vi "final shn 2 .vi"() -> ()   [LabVIEW 2018]
doc: "The myRIO Project template acquires acceleration data from the onboard accelerometer and displays the changes of acceleration values in a waveform chart."
uses:
  <vilib>/myRIO/Instrument Drivers/Onboard IO/DIO/typedefs/DIO Reference.ctl
  <vilib>/myRIO/Common/Instrument Driver Framework/Utilities/typedefs/myRIO Generic Hardware Reference.ctl
  <vilib>/myRIO/Common/Instrument Driver Framework/Utilities/typedefs/Hardware Version Enum.ctl
  <vilib>/myRIO/Common/Instrument Driver Framework/Utilities/typedefs/myRIO v1.0 Reference.ctl
  <vilib>/myRIO/Common/Instrument Driver Framework/Utilities/typedefs/Generic FPGA Reference.ctl
  <vilib>/myRIO/Common/Instrument Driver Framework/myRIO v1.0/DIO/typedefs/DIO Channels List.ctl
  <vilib>/myRIO/Common/Instrument Driver Framework/myRIO v1.0/DIO/typedefs/DIO Channels Enum.ctl
  <vilib>/userdefined/High Color/nirio_resource_hc.ctl
  <vilib>/myRIO/Instrument Drivers/Onboard IO/PWM/typedefs/PWM Reference.ctl
  <vilib>/myRIO/Common/Instrument Driver Framework/myRIO v1.0/PWM/typedefs/PWM Channels Enum.ctl
  <vilib>/myRIO/Instrument Drivers/Onboard IO/PWM/typedefs/PWM Configuration.ctl
  <vilib>/myRIO/Common/Instrument Driver Framework/Utilities/vis/Is FPGA Ref Available.vi
  <vilib>/myRIO/Common/Instrument Driver Framework/myRIO v1.0/DIO/vis/myRIO v1.1 Open DIO.vi
  <vilib>/myRIO/Instrument Drivers/Onboard IO/DIO/vis/Write.vi
  <vilib>/myRIO/Common/Instrument Driver Framework/myRIO v1.0/PWM/vis/myRIO v1.1 Open PWM.vi
  <vilib>/myRIO/Instrument Drivers/Onboard IO/PWM/vis/Set Duty Cycle and Frequency.vi
  <vilib>/myRIO/Common/Instrument Driver Framework/Utilities/vis/Validate Channels.vi
  <vilib>/myRIO/Common/Instrument Driver Framework/myRIO v1.0/DIO/vis/myRIO v1.0 Reserve DIO.vi
  <vilib>/myRIO/Common/Instrument Driver Framework/myRIO v1.0/PWM/vis/myRIO v1.0 Reserve PWM.vi
  <vilib>/myRIO/Common/Instrument Driver Framework/myRIO v1.0/Resource Manager/vis/myRIO v1.0 Reserve Channel List.vi
  <vilib>/myRIO/Common/Instrument Driver Framework/myRIO v1.0/DIO/vis/myRIO v1.0 Build MUX Configuration DIO.vi
  <vilib>/myRIO/Common/Instrument Driver Framework/myRIO v1.0/PWM/vis/myRIO v1.0 Build MUX Configuration PWM.vi
  <vilib>/myRIO/Common/Instrument Driver Framework/myRIO v1.0/Resource Manager/vis/myRIO v1.0 Reserve Channel.vi
  <vilib>/myRIO/Common/Instrument Driver Framework/myRIO v1.0/Resource Manager/vis/myRIO v1.0 Unreserve Channel.vi
  <vilib>/myRIO/Common/Instrument Driver Framework/myRIO v1.0/Resource Manager/vis/myRIO v1.0 Create Configuration List.vi
  <vilib>/myRIO/Common/Instrument Driver Framework/myRIO v1.0/Resource Manager/vis/myRIO v1.0 Build Mutex Name.vi
  <vilib>/Utility/VariantDataType/GetNumericInfo.vi
  <vilib>/Utility/error.llb/Error Cluster From Error Code.vi
  <vilib>/myRIO/Common/Instrument Driver Framework/myRIO v1.0/myRIO v1.1 Open.vi
  <vilib>/myRIO/Common/Instrument Driver Framework/Utilities/vis/IO Manager.vi
  <vilib>/myRIO/Common/Instrument Driver Framework/Utilities/vis/Configuration Manager.vi
  <vilib>/myRIO/Common/Instrument Driver Framework/myRIO v1.0/Resource Manager/vis/myRIO v1.0 Configure IO.vi
  <vilib>/myRIO/Common/Instrument Driver Framework/myRIO v1.0/myRIO v1.0 Close.vi
  <vilib>/myRIO/Common/Instrument Driver Framework/myRIO v1.0/DIO/vis/myRIO v1.0 Write DIO.vi
  <vilib>/myRIO/Common/Instrument Driver Framework/myRIO v1.0/PWM/vis/myRIO v1.0 Write PWM.vi
  <vilib>/myRIO/Express VI/Onboard Devices/LED/LED Express VI.xnode
  <vilib>/myRIO/Instrument Drivers/Onboard IO/DIO/vis/myRIO DIO Open.xnode
  <vilib>/myRIO/Express VI/Onboard IO/PWM/PWM Express VI.xnode
  <vilib>/myRIO/Instrument Drivers/Onboard IO/PWM/vis/myRIO PWM Open.xnode
  <vilib>/myRIO/Express VI/Onboard IO/DO/DO Express VI.xnode
  <vilib>/myRIO/Instrument Drivers/Onboard IO/PWM/PWM.lvlib
  <vilib>/myRIO/Instrument Drivers/Onboard IO/DIO/DIO.lvlib
panel:
  in  "left":bool
  in  "Right":bool
  out "jot connection":bool
  in  "Stop Button 2":bool
  out "message from rio 2":string[](array[string])
  out "Boolean 4":bool=TRUE
  out "Boolean 3":bool=TRUE
  out "Boolean 2":bool
  in  "Stop":bool
  out "Message from Ground Station":string[](array[string])
  in  "horn":bool
  in  "CUTOUT":bool
  in  "Red":bool
  in  "Green":bool
  in  "Yellow":bool
  out "yaw left":bool
  out "yaw right":bool
  out "Duty Cycle 2":dbl=0.5
  out "Duty Cycle":dbl=0.5
  out "thruster 22":dbl
  out "thruster 11":dbl
  out "thruster 2":dbl(slide) scale=0.44..0.76
  out "thruster 1":dbl(slide) scale=0.44..0.76
  out "message from rio":string[](array[string])
  out "surv":dbl
  out "yav":dbl
  out "yad":dbl
  out "surd":dbl
  in  "Stop Button":bool
  out "speed":dbl(slide) scale=0.5..1.0
  out "yaw":dbl(slide) scale=0.0..10000.0
  out "surge":dbl(slide) scale=0.0..10000.0
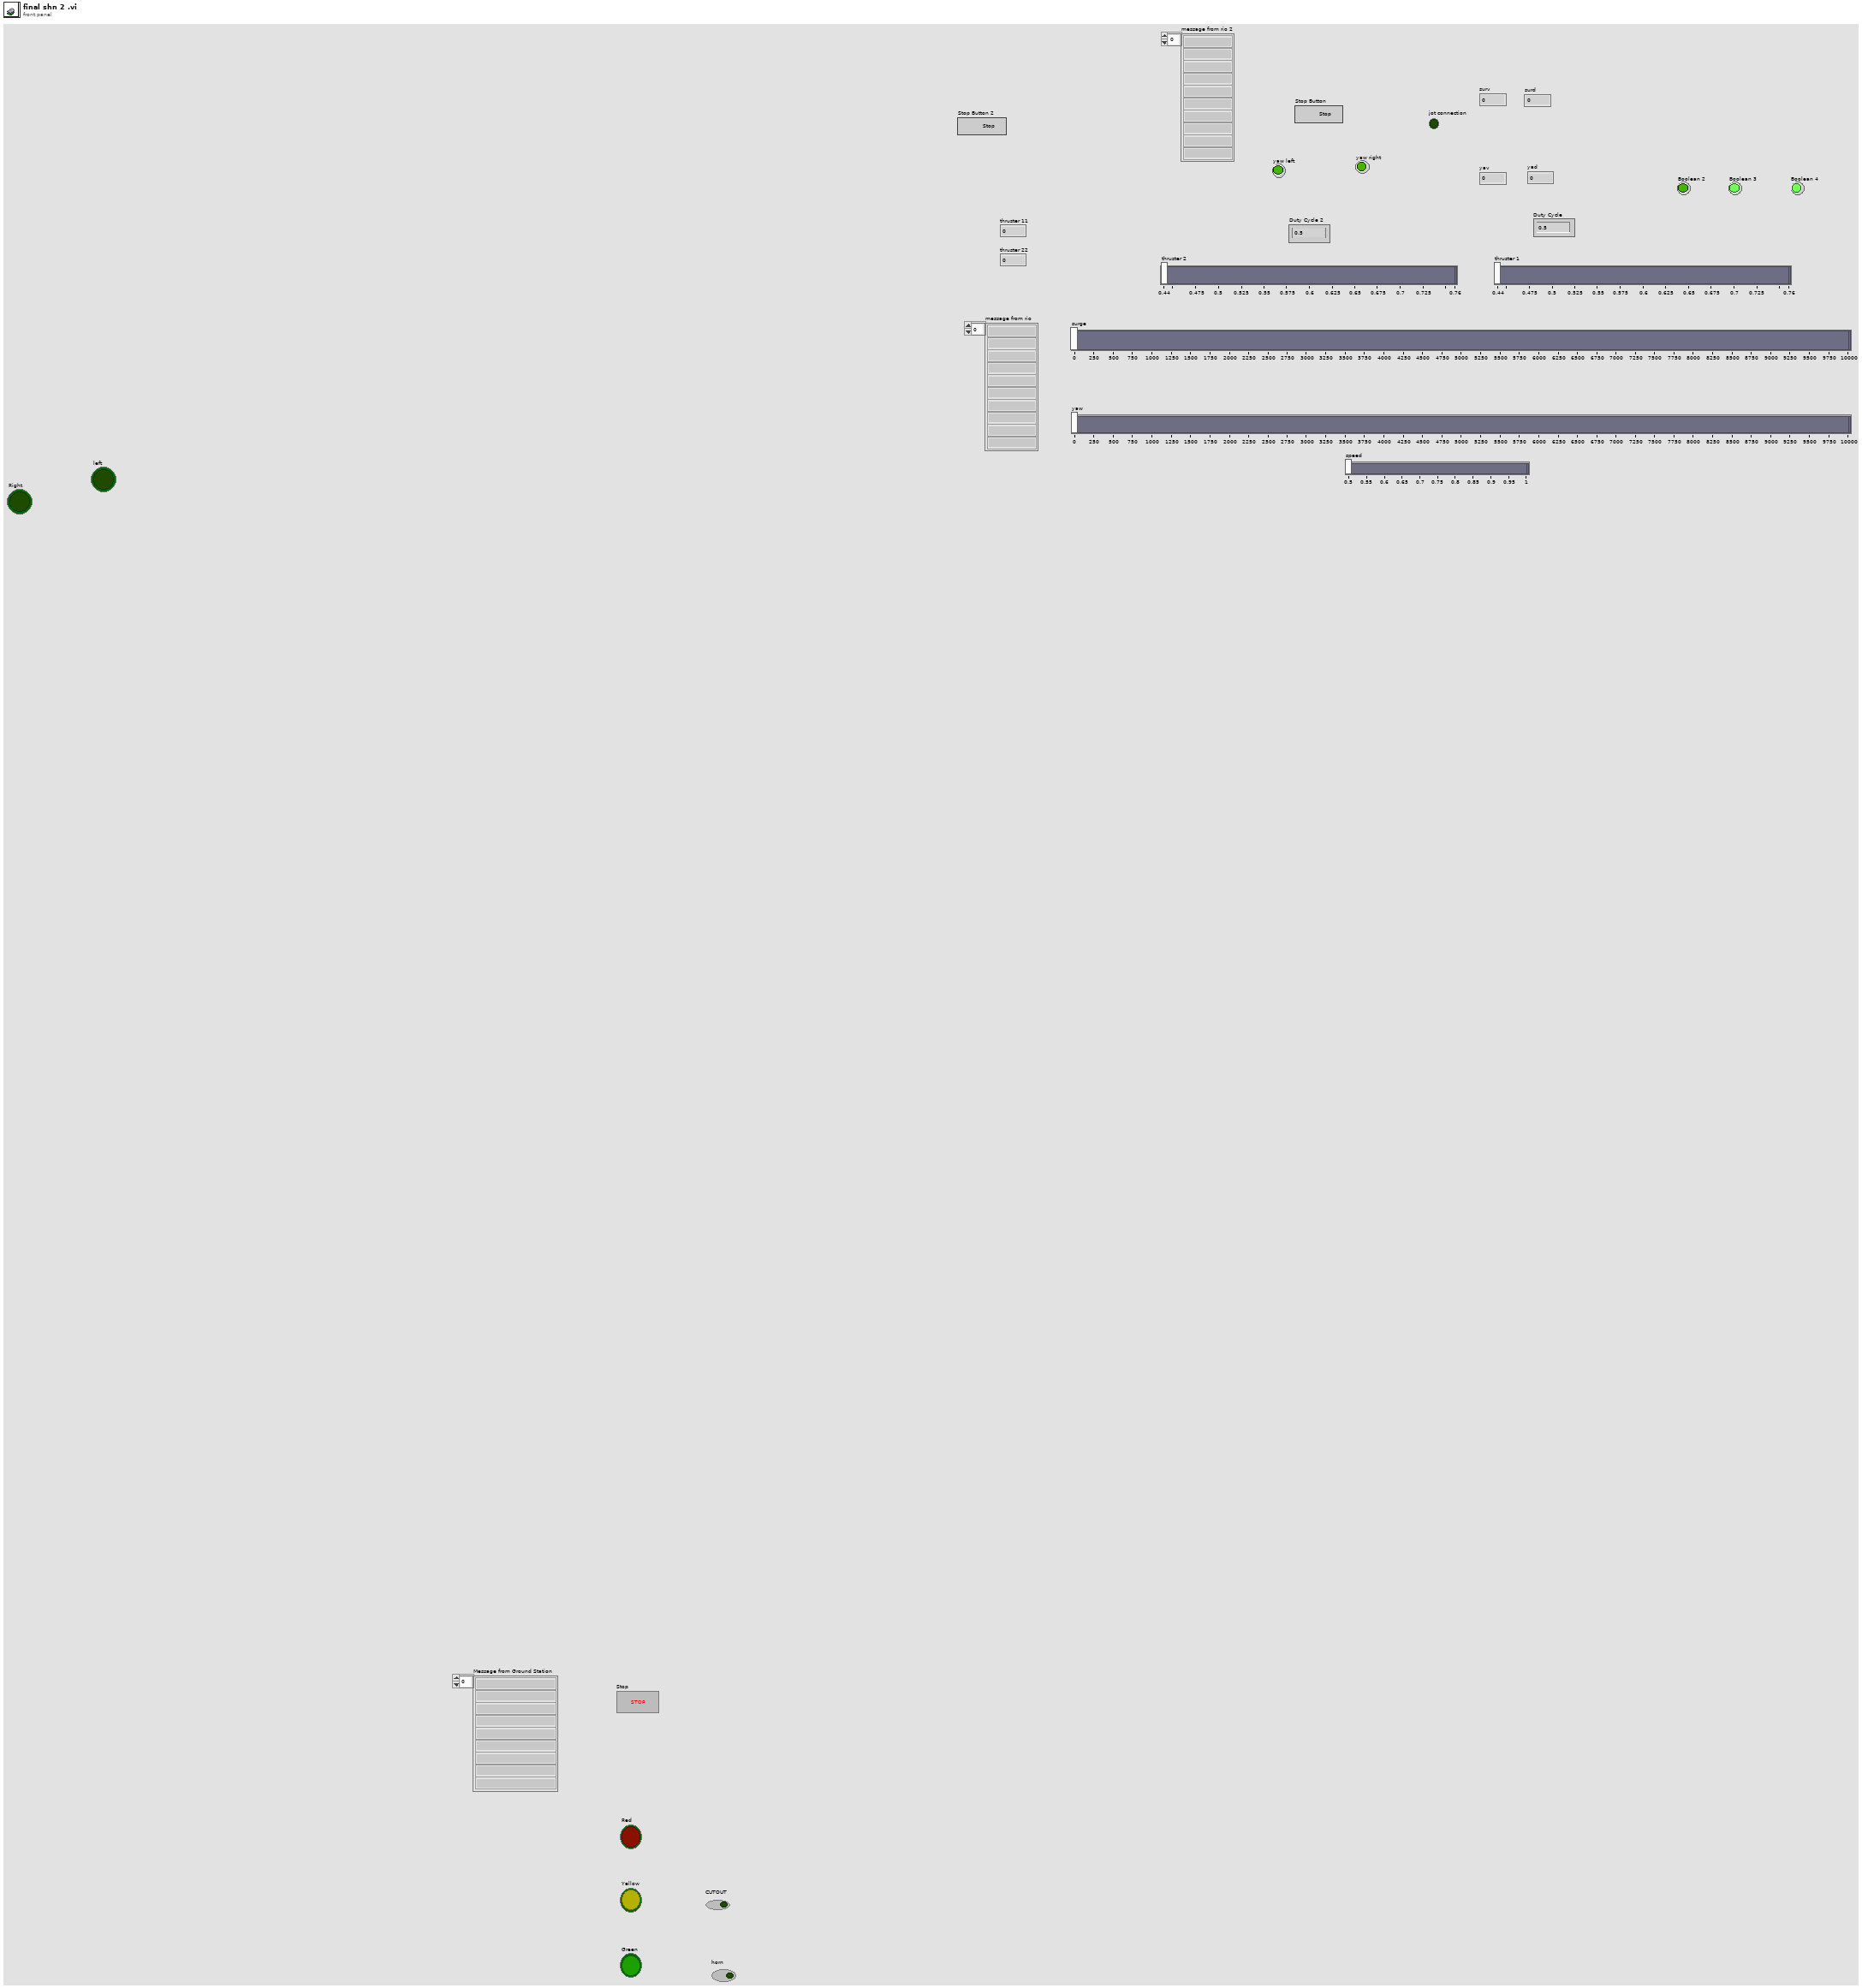
[diagram p1: front panel]
types:
  T1 = typedef "DIO.lvlib/DIO Reference.ctl" = cluster{"myRIO Reference":T2, "DIO Channels List":T6}
  T2 = typedef "myRIO Generic Hardware Reference.ctl" = cluster{"myRIO Model":T3, "myRIO Hardware Reference":T4}
  T3 = typedef "Hardware Version Enum.ctl" = enum16{"Unknown", "myRIO-1900", "myRIO-1950", "roboRIO", "NI ELVIS RIO CM", "ELVIS III"}
  T4 = typedef "myRIO v1.0 Reference.ctl" = cluster{"Generic FPGA Reference":T5, "Allow multiple opens":bool}
  T5 = typedef "Generic FPGA Reference.ctl" = refnum<k20>
  T6 = typedef "DIO Channels List.ctl" = T7[]
  T7 = typedef "DIO Channels Enum.ctl" = enum16{"Not Connected", "C/DIO0", "C/DIO1", "C/DIO2", "C/DIO3", "C/DIO4", "C/DIO5", "C/DIO6", "C/DIO7", "A/DIO0", "A/DIO1", "A/DIO2", "A/DIO3", "A/DIO4", "A/DIO5", "A/DIO6", "A/DIO7", "A/DIO8", "A/DIO9", "A/DIO10", "A/DIO11", "A/DIO12", "A/DIO13", "A/DIO14", "A/DIO15", "A/DIO16", "A/DIO17", "A/DIO18", "A/DIO19", "B/DIO0", "B/DIO1", "B/DIO2", "B/DIO3", "B/DIO4", "B/DIO5", "B/DIO6", "B/DIO7", "B/DIO8", "B/DIO9", "B/DIO10", "B/DIO11", "B/DIO12", "B/DIO13", "B/DIO14", "B/DIO15", "B/DIO16", "B/DIO17", "B/DIO18", "B/DIO19", "LED0", "LED1", "LED2", "LED3", "Button0", "DIO/DIO0", "DIO/DIO1", "DIO/DIO2", "DIO/DIO3", "DIO/DIO4", "DIO/DIO5", "DIO/DIO6", "DIO/DIO7", "DIO/DIO8", "DIO/DIO9", "SPI/CS0", "SPI/CS1", "SPI/CS2", "SPI/CS3", "LED RADIO (Green)", "LED RADIO (Red)", "LED COMM (Green)", "LED COMM (Red)", "LED MODE (Green)", "LED MODE (Red)"}
  T8 = typedef "nirio_resource_hc.ctl" = tag
  T9 = cluster{"[0]":string, "[1]":string, "[2]":string, "[3]":string, "[4]":string, "[5]":string, "[6]":string, "[7]":string, "[8]":string}
  T10 = typedef "PWM.lvlib/PWM Reference.ctl" = cluster{"myRIO Reference":T2, "PWM Channels Enum":T11, "PWM Configuration":T12}
  T11 = typedef "PWM Channels Enum.ctl" = enum16{"Not Connected", "C/PWM0", "C/PWM1", "A/PWM0", "A/PWM1", "A/PWM2", "A/PWM3", "A/PWM4", "A/PWM5", "A/PWM6", "A/PWM7", "A/PWM8", "A/PWM9", "A/PWM10", "A/PWM11", "A/PWM12", "A/PWM13", "A/PWM14", "A/PWM15", "A/PWM16", "A/PWM17", "A/PWM18", "A/PWM19", "B/PWM0", "B/PWM1", "B/PWM2", "B/PWM3", "B/PWM4", "B/PWM5", "B/PWM6", "B/PWM7", "B/PWM8", "B/PWM9", "B/PWM10", "B/PWM11", "B/PWM12", "B/PWM13", "B/PWM14", "B/PWM15", "B/PWM16", "B/PWM17", "B/PWM18", "B/PWM19", "PWM/PWM0", "PWM/PWM1", "PWM/PWM2", "PWM/PWM3", "PWM/PWM4", "PWM/PWM5", "PWM/PWM6", "PWM/PWM7", "PWM/PWM8", "PWM/PWM9"}
  T12 = typedef "PWM.lvlib/PWM Configuration.ctl" = cluster{"Frequency":dbl, "Duty Cycle":dbl}
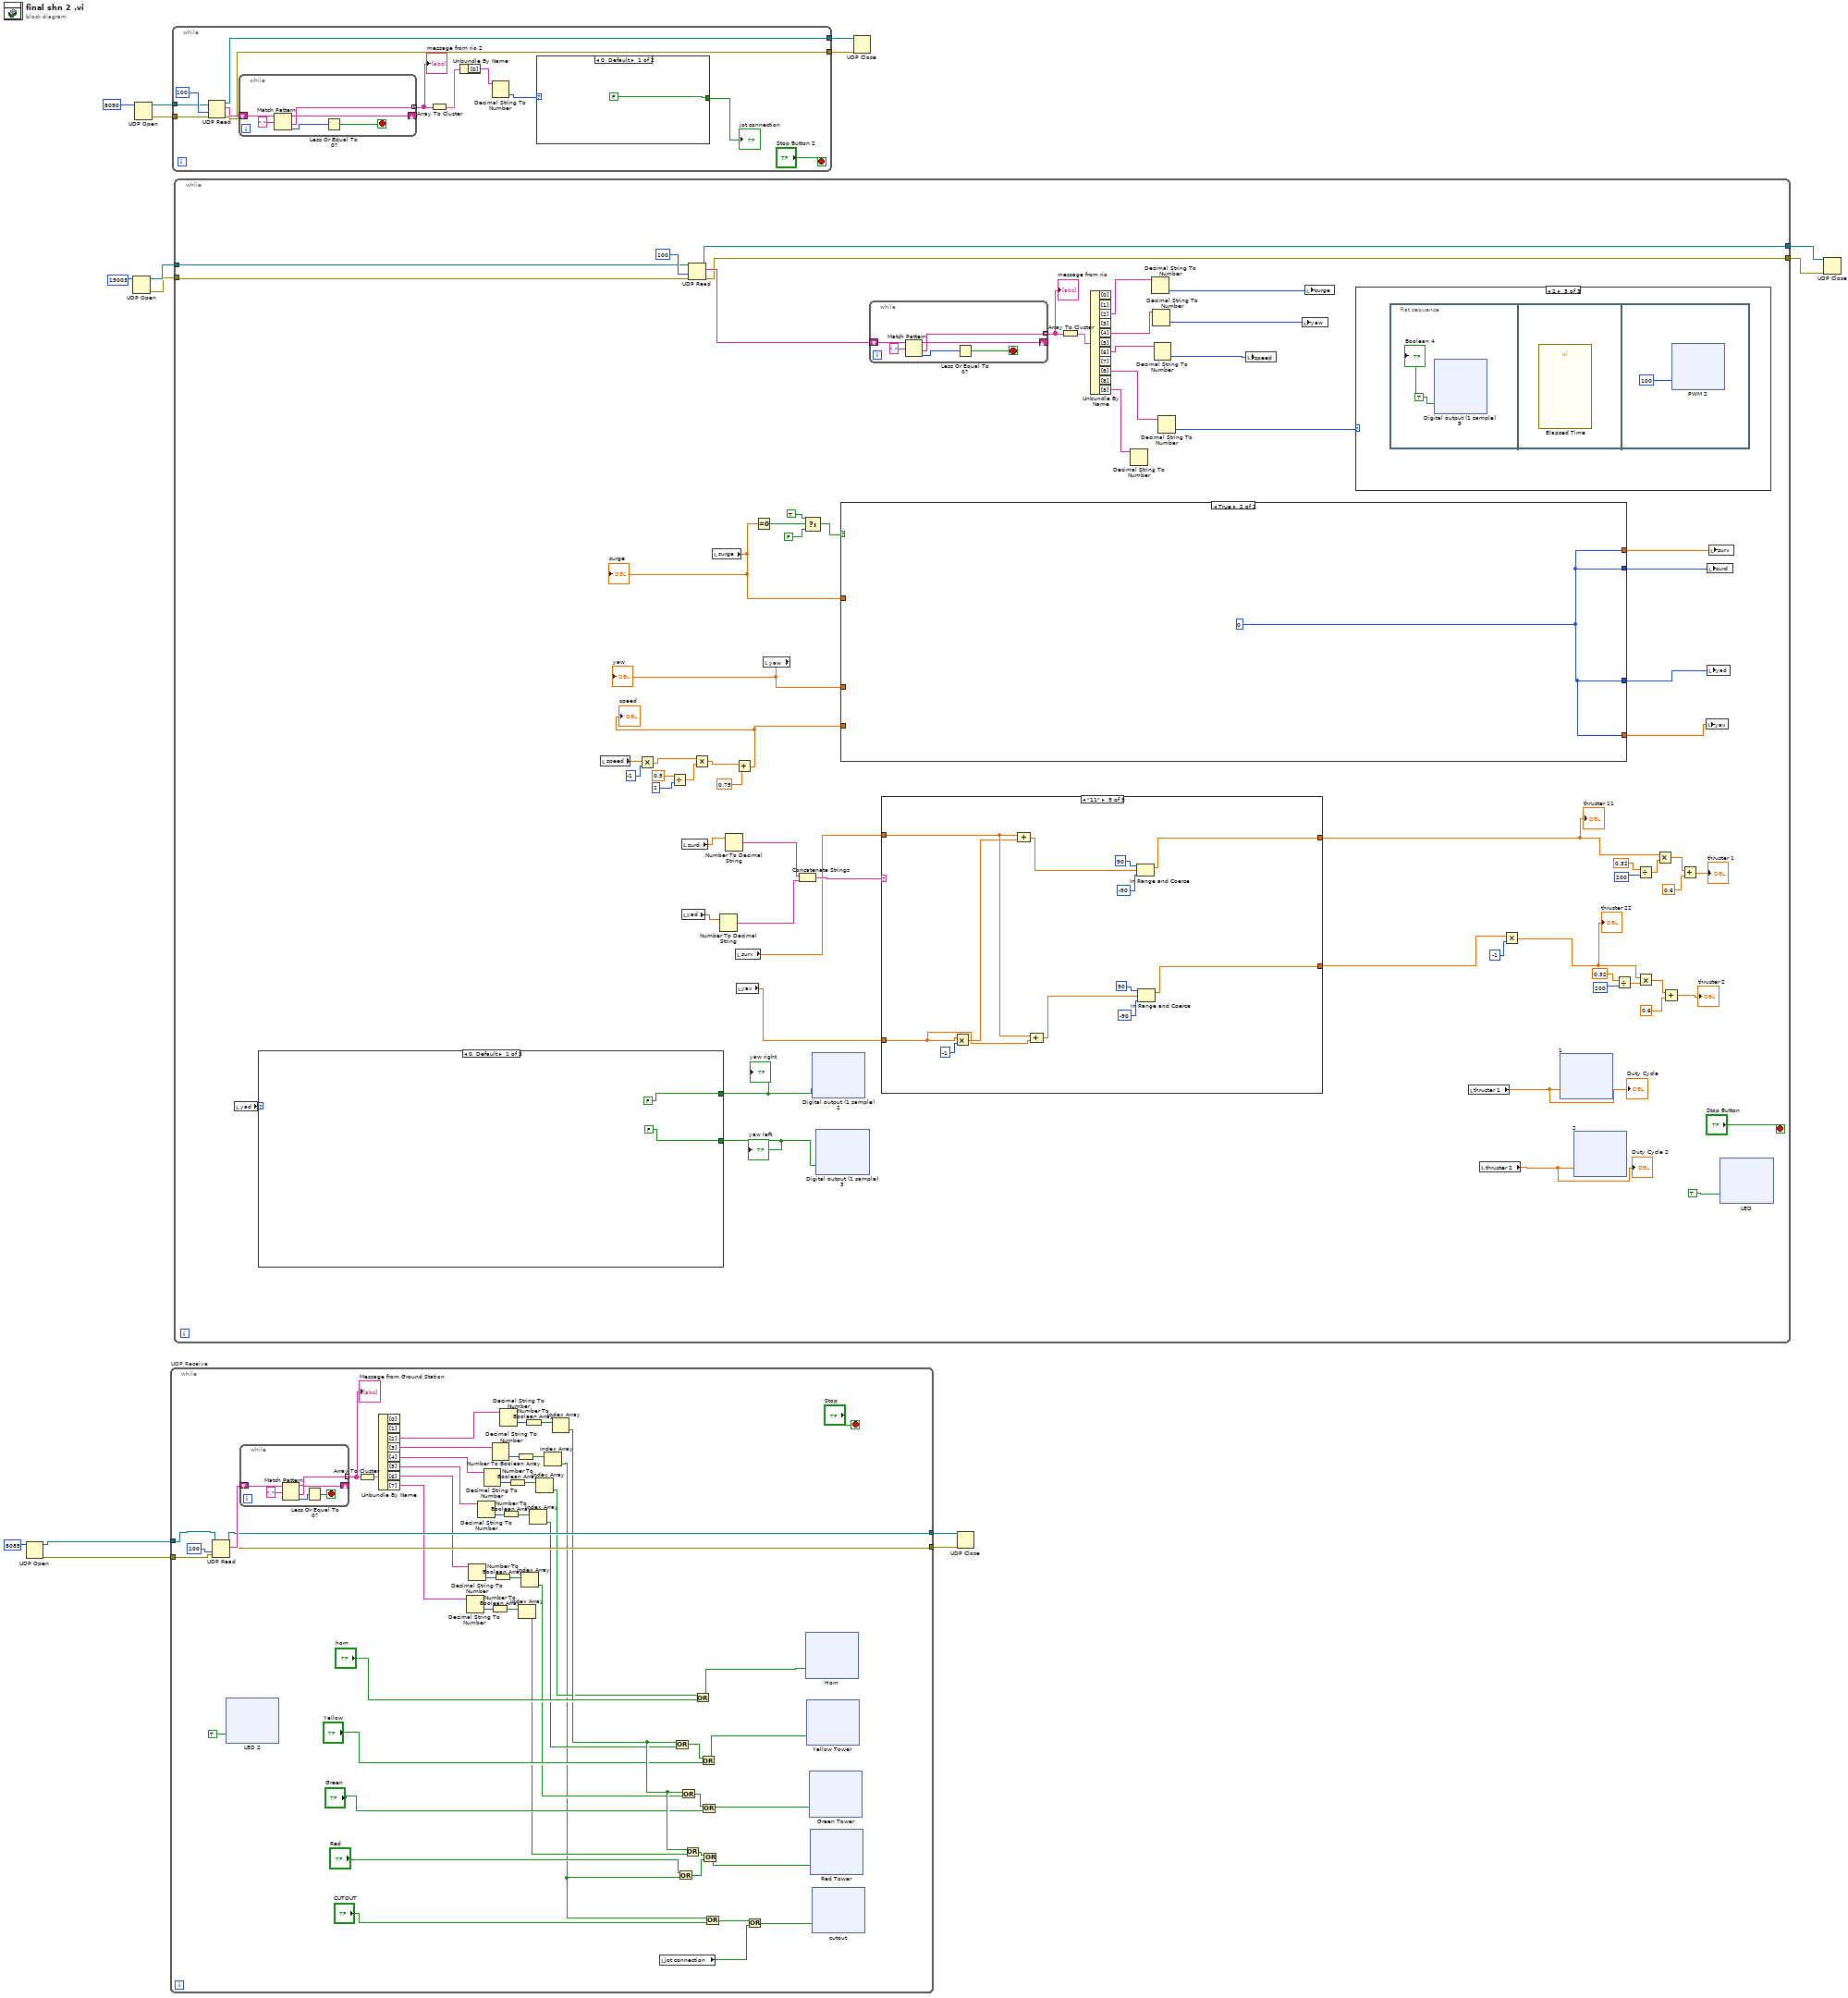
[diagram p0: block diagram]
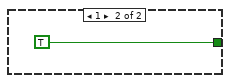
[diagram p2: hidden frame]
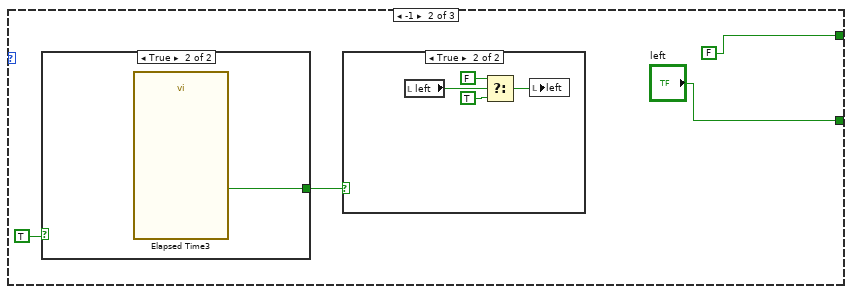
[diagram p3: hidden frame]
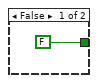
[diagram p4: hidden frame]
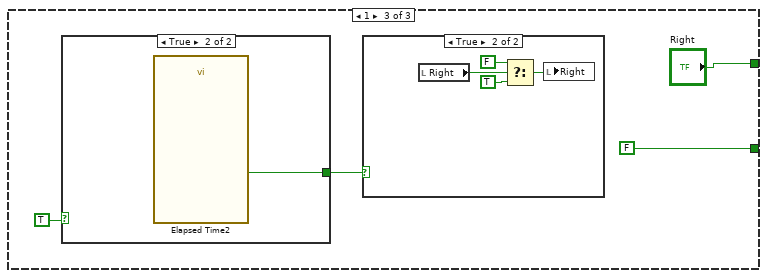
[diagram p6: hidden frame]
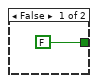
[diagram p7: hidden frame]
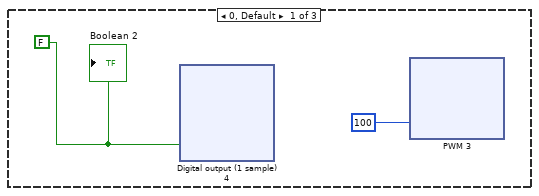
[diagram p9: hidden frame]
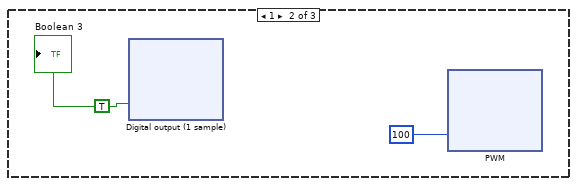
[diagram p10: hidden frame]
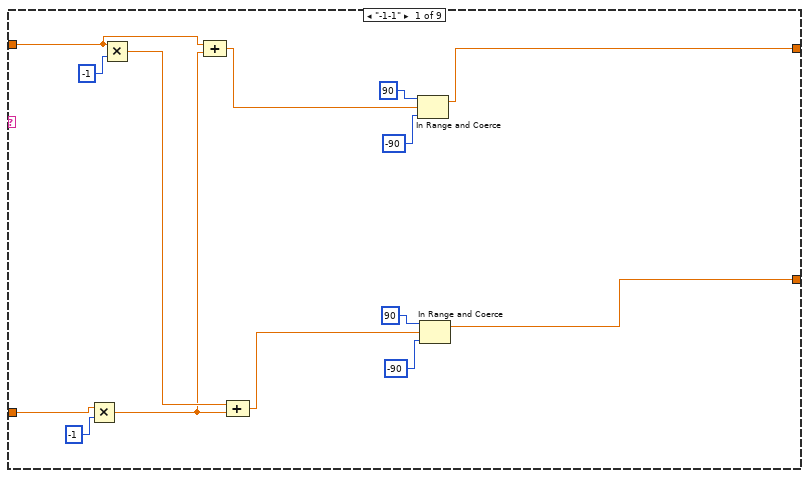
[diagram p11: hidden frame]
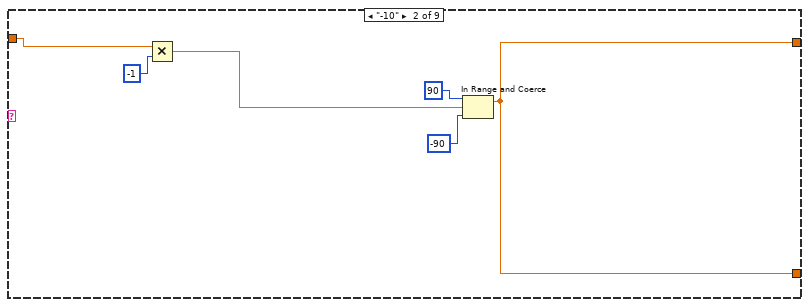
[diagram p12: hidden frame]
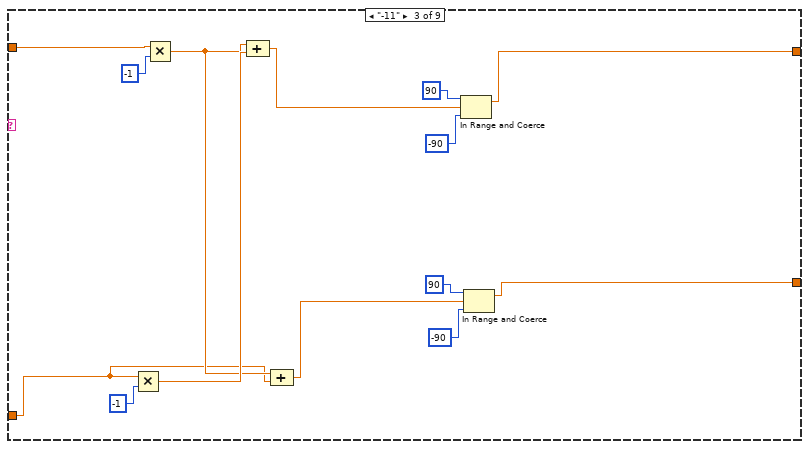
[diagram p13: hidden frame]
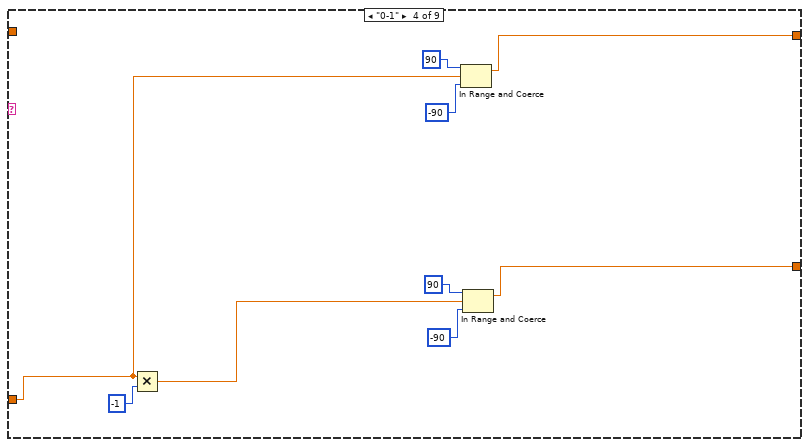
[diagram p14: hidden frame]
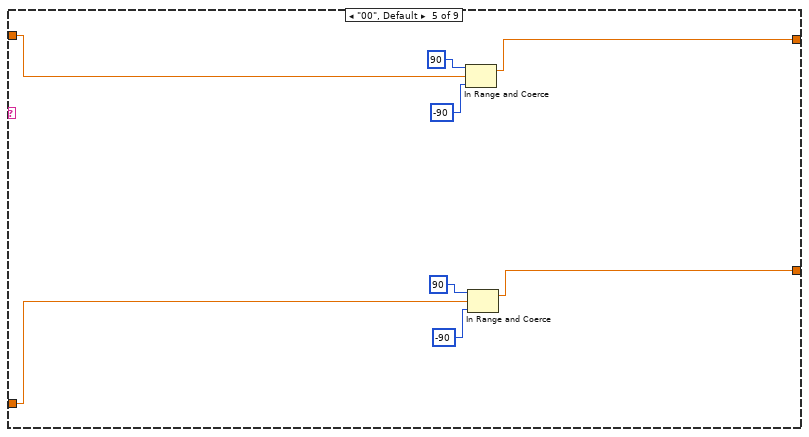
[diagram p15: hidden frame]
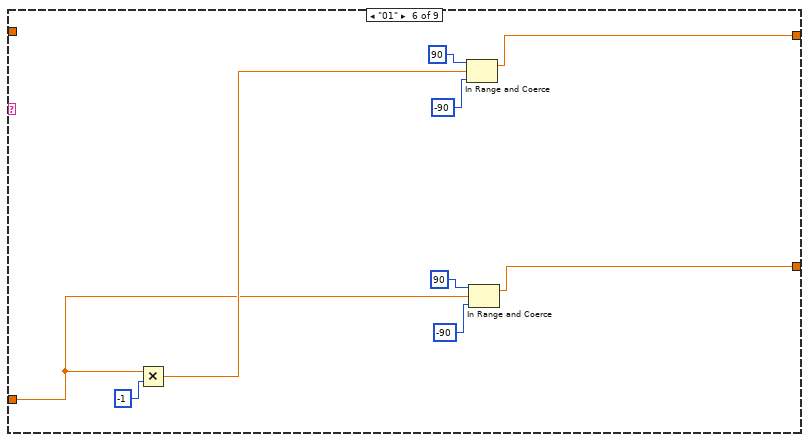
[diagram p16: hidden frame]
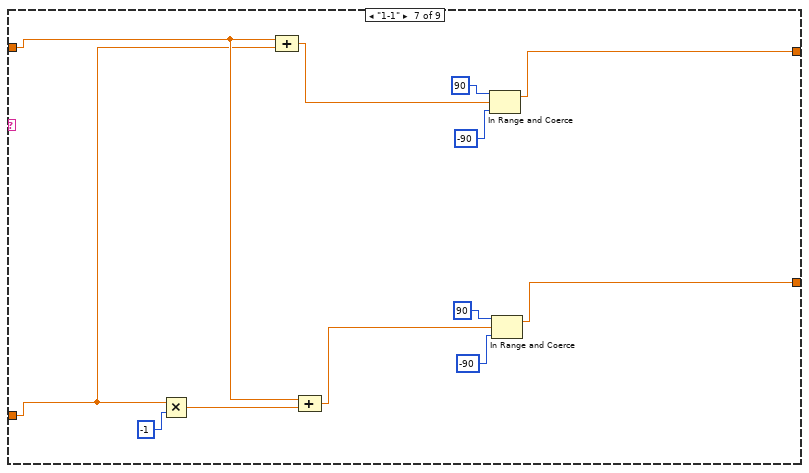
[diagram p17: hidden frame]
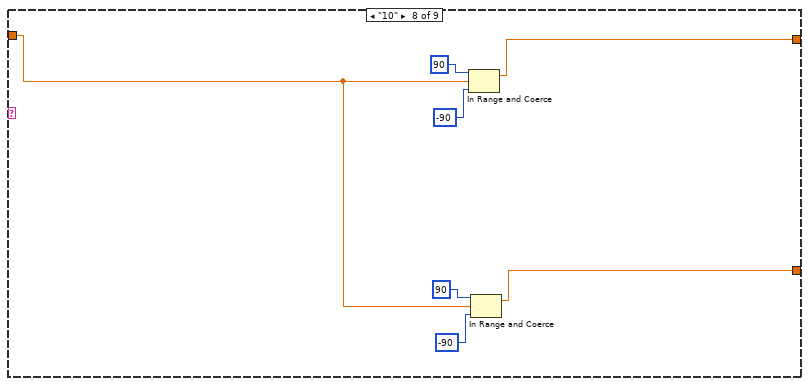
[diagram p18: hidden frame]
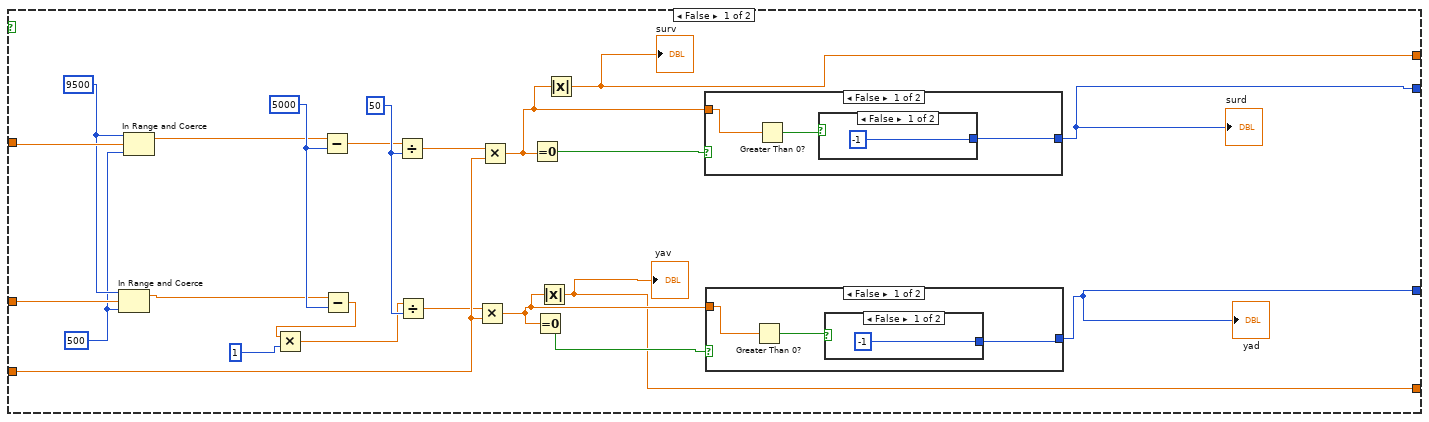
[diagram p19: hidden frame]
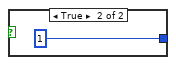
[diagram p20: hidden frame]
diagram:
  n1 = UDP Open(11:u16 8085 ("port")) -> (port=w9:refnum<k16>, 0:w8:errorcluster)  [unwired: 4 in, 1 out]
  n2 = UDP Open(11:u16 15003 ("port")) -> (port=w14:refnum<k16>, 0:w13:errorcluster)  [unwired: 4 in, 1 out]
  n3 = UDP Open(11:u16 8090 ("port")) -> (port=w4:refnum<k16>, 0:w3:errorcluster)  [unwired: 4 in, 1 out]
  n4 = while "UDP Receive" {
    tunnel: [w64] -> w7
    tunnel: [w63] -> w6
    tunnel: w9 -> [w25]
    tunnel: w8 -> [w24]
    stop <- "Stop" stop-if-true
    n5 = UDP Read(connection ID=w25, timeout ms (25000)=100, 8:w24) -> (data out=w65:string, error out=w63:errorcluster, 3:w64:refnum<k16>)  [unwired: 1 in, 2 out]
    n6 = xnode "LED 2"("LED3"=TRUE) -> ()  [unwired: 1 in, 1 out]
    n7 = while {
      tunnel: [w278] -> w60 mode=indexing
      shift-right: [w279] -> _
      shift-left: w65 -> [w281]
      stop <- w276 stop-if-true
      n8 = Match Pattern(string=w281, regular expression=",") -> (before substring=w278:string, after substring=w279:string, offset past match=w277:i32)  [unwired: 1 in, 1 out]
      n9 = Less Or Equal To 0?(x=w277) -> (x <= 0?=w276:bool)
    }
    "Message from Ground Station" <- w60
    n10 = Array To Cluster(array=w60) -> (cluster=w61:T9)
    n11 = Unbundle By Name(w61) -> ("[2]"=w49:string, "[3]"=w48:string, "[4]"=w45:string, "[5]"=w42:string, "[6]"=w39:string, "[7]"=w36:string)  [unwired: 2 out]
    n12 = Decimal String To Number(string=w36) -> (number=w37:i32)  [unwired: 2 in, 1 out]
    n13 = Decimal String To Number(string=w39) -> (number=w41:i32)  [unwired: 2 in, 1 out]
    n14 = Decimal String To Number(string=w42) -> (number=w43:i32)  [unwired: 2 in, 1 out]
    n15 = Decimal String To Number(string=w45) -> (number=w47:i32)  [unwired: 2 in, 1 out]
    n16 = Decimal String To Number(string=w48) -> (number=w50:i32)  [unwired: 2 in, 1 out]
    n17 = Number To Boolean Array(number=w37) -> (Boolean array=w38:bool[])
    n18 = Number To Boolean Array(number=w41) -> (Boolean array=w40:bool[])
    n19 = Decimal String To Number(string=w49) -> (number=w59:i32)  [unwired: 2 in, 1 out]
    n20 = Number To Boolean Array(number=w43) -> (Boolean array=w44:bool[])
    n21 = Number To Boolean Array(number=w47) -> (Boolean array=w46:bool[])
    n22 = Number To Boolean Array(number=w50) -> (Boolean array=w51:bool[])
    n23 = Index Array(array=w38) -> (element=w30:bool)  [unwired: 1 in]
    n24 = Index Array(array=w40) -> (element=w31:bool)  [unwired: 1 in]
    n25 = Number To Boolean Array(number=w59) -> (Boolean array=w58:bool[])
    n26 = Index Array(array=w44) -> (element=w32:bool)  [unwired: 1 in]
    n27 = Index Array(array=w46) -> (element=w33:bool)  [unwired: 1 in]
    n28 = Index Array(array=w51) -> (element=w26:bool)  [unwired: 1 in]
    n29 = Index Array(array=w58) -> (element=w52:bool)  [unwired: 1 in]
    n30 = local read "jot connection"() -> (w18:bool)
    n31 = Or(x=w52, y=w32) -> (x .or. y?=w55:bool)
    n32 = Or(x="Red", y=w26) -> (x .or. y?=w27:bool)
    n33 = Or(x=w52, y=w31) -> (x .or. y?=w53:bool)
    n34 = Or(x=w52, y=w30) -> (x .or. y?=w54:bool)
    n35 = Or(x=w33, y="horn") -> (x .or. y?=w23:bool)
    n36 = Or(x=w55, y="Yellow") -> (x .or. y?=w22:bool)
    n37 = Or(x=w53, y="Green") -> (x .or. y?=w21:bool)
    n38 = Or(x=w54, y=w27) -> (x .or. y?=w20:bool)
    n39 = Or(x=w26, y="CUTOUT") -> (x .or. y?=w17:bool)
    n40 = Or(x=w17, y=w18) -> (x .or. y?=w16:bool)
    n41 = xnode "Horn"("A/DIO3 (Pin 17)"=w23) -> ()  [unwired: 1 in, 1 out]
    n42 = xnode "Yellow Tower"("A/DIO4 (Pin 19)"=w22) -> ()  [unwired: 1 in, 1 out]
    n43 = xnode "Green Tower"("A/DIO5 (Pin 21)"=w21) -> ()  [unwired: 1 in, 1 out]
    n44 = xnode "Red Tower"("A/DIO6 (Pin 23)"=w20) -> ()  [unwired: 1 in, 1 out]
    n45 = xnode "cutout"("A/DIO7 (Pin 25)"=w16) -> ()  [unwired: 1 in, 1 out]
  }
  n46 = while {
    tunnel: w4 -> [w290]
    tunnel: w3 -> [w289]
    tunnel: [w284] -> w2
    tunnel: [w283] -> w1
    stop <- "Stop Button 2" stop-if-true
    n47 = UDP Read(connection ID=w290, timeout ms (25000)=100, 8:w289) -> (data out=w285:string, error out=w283:errorcluster, 3:w284:refnum<k16>)  [unwired: 1 in, 2 out]
    n48 = while {
      tunnel: [w298] -> w292 mode=indexing
      shift-right: [w299] -> _
      shift-left: w285 -> [w301]
      stop <- w296 stop-if-true
      n49 = Match Pattern(string=w301, regular expression=",") -> (before substring=w298:string, after substring=w299:string, offset past match=w297:i32)  [unwired: 1 in, 1 out]
      n50 = Less Or Equal To 0?(x=w297) -> (x <= 0?=w296:bool)
    }
    "message from rio 2" <- w292
    n51 = Array To Cluster(array=w292) -> (cluster=w293:T9)
    n52 = Unbundle By Name(w293) -> ("[0]"=w288:string)
    n53 = Decimal String To Number(string=w288) -> (number=w287:i32)  [unwired: 2 in, 1 out]
    n54 = case shown="0, Default" w287 {
      tunnel: [FALSE TRUE] -> w282
      frame 0, Default {
      }
      frame 1 {
      }
    }
    "jot connection" <- w282
  }
  n55 = while {
    tunnel: [w341] -> w12
    tunnel: w14 -> [w340]
    tunnel: w13 -> [w339]
    tunnel: [w324] -> w11
    stop <- "Stop Button" stop-if-true
    n56 = local read "yad"() -> (w302:dbl)
    n57 = case shown="0, Default" w302 {
      tunnel: [FALSE FALSE "Right"] -> w303
      tunnel: [FALSE "left" FALSE] -> w307
      frame 0, Default {
      }
      frame -1 {
        n58 = case shown="True" TRUE {
          tunnel: [FALSE ("Time has Elapsed") w375] -> w372
          frame False {
          }
          frame True {
            n59 = call "Elapsed Time3"() -> ("Time has Elapsed"=w375:bool)  [unwired: 12 in, 7 out]
          }
        }
        n60 = case shown="True" w372 {
          frame False {
          }
          frame True {
            n61 = local read "left"() -> (w376:bool)
            n62 = Select(t=FALSE, s=w376, f=TRUE) -> (s? t:f=w377:bool)
            n63 = local write "left"(w377) -> ()
          }
        }
      }
      frame 1 {
        n64 = case shown="True" TRUE {
          tunnel: [FALSE ("Time has Elapsed") w385] -> w382
          frame False {
          }
          frame True {
            n65 = call "Elapsed Time2"() -> ("Time has Elapsed"=w385:bool)  [unwired: 12 in, 7 out]
          }
        }
        n66 = case shown="True" w382 {
          frame False {
          }
          frame True {
            n67 = local read "Right"() -> (w386:bool)
            n68 = Select(t=FALSE, s=w386, f=TRUE) -> (s? t:f=w387:bool)
            n69 = local write "Right"(w387) -> ()
          }
        }
      }
    }
    "yaw right" <- w303
    "yaw left" <- w307
    n70 = local read "speed"() -> (w332:dbl)
    n71 = Multiply(x=w332, y=-1) -> (x*y=w328:dbl)
    n72 = Divide(x=0.5, y=2) -> (x/y=w327:dbl)
    n73 = local read "yad"() -> (w360:dbl)
    n74 = local read "surd"() -> (w361:dbl)
    n75 = UDP Read(connection ID=w340, timeout ms (25000)=100, 8:w339) -> (data out=w345:string, error out=w341:errorcluster, 3:w324:refnum<k16>)  [unwired: 1 in, 2 out]
    n76 = Multiply(x=w328, y=w327) -> (x*y=w326:dbl)
    n77 = local read "surge"() -> (w333:dbl)
    "surge" <- w333
    n78 = Number To Decimal String(number=w360) -> (decimal integer string=w318:string)  [unwired: 1 in]
    n79 = Number To Decimal String(number=w361) -> (decimal integer string=w362:string)  [unwired: 1 in]
    n80 = Add(x=w326, y=0.75) -> (x+y=w306:dbl)
    "speed" <- w306
    n81 = local read "surv"() -> (w316:dbl)
    n82 = local read "yav"() -> (w315:dbl)
    n83 = Equal To 0?(x=w333) -> (x = 0?=w367:bool)
    n84 = local read "yaw"() -> (w334:dbl)
    "yaw" <- w334
    n85 = Concatenate Strings(w362, w318) -> (w317:string)
    n86 = Select(t=TRUE, s=w367, f=FALSE) -> (s? t:f=w366:bool)
    n87 = xnode "Digital output (1 sample) 2"("A/DIO1 (Pin 13)"=w303) -> ()  [unwired: 1 in, 1 out]
    n88 = xnode "Digital output (1 sample) 3"("A/DIO2 (Pin 15)"=w307) -> ()  [unwired: 1 in, 1 out]
    n89 = case shown="True" w366 {
      tunnel: w334 -> [w896 _]
      tunnel: w306 -> [w891 _]
      tunnel: w333 -> [w897 _]
      tunnel: [w884 w913] -> w359
      tunnel: [w883 w913] -> w358
      tunnel: [w882 w913] -> w357
      tunnel: [w881 w913] -> w356
      frame False {
        w894 = 500
        w895 = 9500
        w899 = 50
        w900 = 5000
        n90 = In Range and Coerce(upper limit=w895, x=w896, lower limit=w894) -> (coerced(x)=w892:dbl)  [unwired: 1 out]
        n91 = In Range and Coerce(upper limit=w895, x=w897, lower limit=w894) -> (coerced(x)=w893:dbl)  [unwired: 1 out]
        n92 = Subtract(x=w893, y=w900) -> (x-y=w898:dbl)
        n93 = Subtract(x=w892, y=w900) -> (x-y=w879:dbl)
        n94 = Multiply(x=w879, y=1) -> (x*y=w878:dbl)
        n95 = Divide(x=w898, y=w899) -> (x/y=w890:dbl)
        n96 = Divide(x=w878, y=w899) -> (x/y=w889:dbl)
        n97 = Multiply(x=w889, y=w891) -> (x*y=w885:dbl)
        n98 = Multiply(x=w890, y=w891) -> (x*y=w886:dbl)
        n99 = Equal To 0?(x=w886) -> (x = 0?=w888:bool)
        n100 = Equal To 0?(x=w885) -> (x = 0?=w887:bool)
        n101 = Absolute Value(x=w885) -> (abs(x)=w881:dbl)
        "yav" <- w881
        n102 = Absolute Value(x=w886) -> (abs(x)=w882:dbl)
        "surv" <- w882
        n103 = case shown="False" w888 {
          tunnel: [w907 0] -> w883
          tunnel: w886 -> [w909 _]
          frame False {
            n104 = Greater Than 0?(x=w909) -> (x > 0?=w908:bool)
            n105 = case shown="False" w908 {
              tunnel: [-1 1] -> w907
              frame False {
              }
              frame True {
              }
            }
          }
          frame True {
          }
        }
        "surd" <- w883
        n106 = case shown="False" w887 {
          tunnel: w885 -> [w903 _]
          tunnel: [w901 0] -> w884
          frame False {
            n107 = Greater Than 0?(x=w903) -> (x > 0?=w902:bool)
            n108 = case shown="False" w902 {
              tunnel: [-1 1] -> w901
              frame False {
              }
              frame True {
              }
            }
          }
          frame True {
          }
        }
        "yad" <- w884
      }
      frame True {
        w913 = 0
      }
    }
    n109 = while {
      tunnel: [w874] -> w343 mode=indexing
      shift-right: [w875] -> _
      shift-left: w345 -> [w877]
      stop <- w872 stop-if-true
      n110 = Match Pattern(string=w877, regular expression=",") -> (before substring=w874:string, after substring=w875:string, offset past match=w873:i32)  [unwired: 1 in, 1 out]
      n111 = Less Or Equal To 0?(x=w873) -> (x <= 0?=w872:bool)
    }
    "message from rio" <- w343
    n112 = case shown="\"11\"" w317 {
      tunnel: w316 -> [w678 w692 w703 _ w722 _ w740 w750 w759]
      tunnel: w315 -> [w681 _ w696 w711 w721 w727 w737 _ w755]
      tunnel: [w682 w690 w701 w713 w720 w730 w741 w749 w760] -> w314
      tunnel: [w679 w690 w699 w712 w719 w729 w738 w748 w757] -> w312
      frame "-1-1" {
        n113 = Multiply(x=w681, y=-1) -> (x*y=w676:dbl)
        n114 = Multiply(x=w678, y=-1) -> (x*y=w677:dbl)
        n115 = Compound Arithmetic op=ADD(w678, w676) -> (w683:dbl)
        n116 = Compound Arithmetic op=ADD(w677, w676) -> (w680:dbl)
        n117 = In Range and Coerce(upper limit=90, x=w683, lower limit=-90) -> (coerced(x)=w682:dbl)  [unwired: 1 out]
        n118 = In Range and Coerce(upper limit=90, x=w680, lower limit=-90) -> (coerced(x)=w679:dbl)  [unwired: 1 out]
      }
      frame "-10" {
        n119 = Multiply(x=w692, y=-1) -> (x*y=w691:dbl)
        n120 = In Range and Coerce(upper limit=90, x=w691, lower limit=-90) -> (coerced(x)=w690:dbl)  [unwired: 1 out]
      }
      frame "-11" {
        n121 = Multiply(x=w696, y=-1) -> (x*y=w698:dbl)
        n122 = Multiply(x=w703, y=-1) -> (x*y=w697:dbl)
        n123 = Compound Arithmetic op=ADD(w697, w698) -> (w702:dbl)
        n124 = Compound Arithmetic op=ADD(w697, w696) -> (w700:dbl)
        n125 = In Range and Coerce(upper limit=90, x=w702, lower limit=-90) -> (coerced(x)=w701:dbl)  [unwired: 1 out]
        n126 = In Range and Coerce(upper limit=90, x=w700, lower limit=-90) -> (coerced(x)=w699:dbl)  [unwired: 1 out]
      }
      frame "0-1" {
        n127 = Multiply(x=w711, y=-1) -> (x*y=w710:dbl)
        n128 = In Range and Coerce(upper limit=90, x=w711, lower limit=-90) -> (coerced(x)=w713:dbl)  [unwired: 1 out]
        n129 = In Range and Coerce(upper limit=90, x=w710, lower limit=-90) -> (coerced(x)=w712:dbl)  [unwired: 1 out]
      }
      frame "00", Default {
        n130 = In Range and Coerce(upper limit=90, x=w722, lower limit=-90) -> (coerced(x)=w720:dbl)  [unwired: 1 out]
        n131 = In Range and Coerce(upper limit=90, x=w721, lower limit=-90) -> (coerced(x)=w719:dbl)  [unwired: 1 out]
      }
      frame "01" {
        n132 = Multiply(x=w727, y=-1) -> (x*y=w728:dbl)
        n133 = In Range and Coerce(upper limit=90, x=w728, lower limit=-90) -> (coerced(x)=w730:dbl)  [unwired: 1 out]
        n134 = In Range and Coerce(upper limit=90, x=w727, lower limit=-90) -> (coerced(x)=w729:dbl)  [unwired: 1 out]
      }
      frame "1-1" {
        n135 = Multiply(x=w737, y=-1) -> (x*y=w736:dbl)
        n136 = Compound Arithmetic op=ADD(w740, w737) -> (w742:dbl)
        n137 = Compound Arithmetic op=ADD(w740, w736) -> (w739:dbl)
        n138 = In Range and Coerce(upper limit=90, x=w742, lower limit=-90) -> (coerced(x)=w741:dbl)  [unwired: 1 out]
        n139 = In Range and Coerce(upper limit=90, x=w739, lower limit=-90) -> (coerced(x)=w738:dbl)  [unwired: 1 out]
      }
      frame "10" {
        n140 = In Range and Coerce(upper limit=90, x=w750, lower limit=-90) -> (coerced(x)=w749:dbl)  [unwired: 1 out]
        n141 = In Range and Coerce(upper limit=90, x=w750, lower limit=-90) -> (coerced(x)=w748:dbl)  [unwired: 1 out]
      }
      frame "11" {
        n142 = Multiply(x=w755, y=-1) -> (x*y=w756:dbl)
        n143 = Compound Arithmetic op=ADD(w759, w756) -> (w761:dbl)
        n144 = Compound Arithmetic op=ADD(w759, w755) -> (w758:dbl)
        n145 = In Range and Coerce(upper limit=90, x=w761, lower limit=-90) -> (coerced(x)=w760:dbl)  [unwired: 1 out]
        n146 = In Range and Coerce(upper limit=90, x=w758, lower limit=-90) -> (coerced(x)=w757:dbl)  [unwired: 1 out]
      }
    }
    "thruster 11" <- w314
    n147 = Array To Cluster(array=w343) -> (cluster=w344:T9)
    n148 = Unbundle By Name(w344) -> ("[2]"=w338:string, "[4]"=w337:string, "[6]"=w336:string, "[8]"=w335:string, "[8]"=w310:string)  [unwired: 6 out]
    n149 = Decimal String To Number(string=w310) -> ()  [unwired: 2 in, 2 out]
    n150 = Decimal String To Number(string=w338) -> (number=w309:i32)  [unwired: 2 in, 1 out]
    n151 = Decimal String To Number(string=w337) -> (number=w308:i32)  [unwired: 2 in, 1 out]
    n152 = Decimal String To Number(string=w336) -> (number=w305:i32)  [unwired: 2 in, 1 out]
    n153 = Decimal String To Number(string=w335) -> (number=w304:i32)  [unwired: 2 in, 1 out]
    n154 = local write "speed"(w305) -> ()
    n155 = local write "yaw"(w308) -> ()
    n156 = local write "surge"(w309) -> ()
    n157 = case shown="2" w304 {
      frame 0, Default {
        w461 = FALSE
        n158 = xnode "Digital output (1 sample) 4"("A/DIO0 (Pin 11)"=w461) -> ()  [unwired: 1 in, 1 out]
        n159 = xnode "PWM 3"("Duty Cycle"=100) -> ()  [unwired: 1 in, 1 out]
        "Boolean 2" <- w461
      }
      frame 1 {
        w532 = TRUE
        n160 = xnode "Digital output (1 sample)"("A/DIO0 (Pin 11)"=w532) -> ()  [unwired: 1 in, 1 out]
        n161 = xnode "PWM"("Duty Cycle"=100) -> ()  [unwired: 1 in, 1 out]
        "Boolean 3" <- w532
      }
      frame 2 {
        n162 = flat-sequence {
          frame #0 {
            w604 = TRUE
            n163 = xnode "Digital output (1 sample) 5"("A/DIO0 (Pin 11)"=w604) -> ()  [unwired: 1 in, 1 out]
            "Boolean 4" <- w604
          }
          frame #1 {
            n164 = call "Elapsed Time"() -> ()  [unwired: 12 in, 8 out]
          }
          frame #2 {
            n165 = xnode "PWM 2"("Duty Cycle"=100) -> ()  [unwired: 1 in, 1 out]
          }
        }
      }
    }
    n166 = local read "thruster 1"() -> (w320:dbl)
    "Duty Cycle" <- w320
    n167 = local read "thruster 2"() -> (w319:dbl)
    "Duty Cycle 2" <- w319
    n168 = Multiply(x=w312, y=-1) -> (x*y=w311:dbl)
    "thruster 22" <- w311
    n169 = xnode "1"("Duty Cycle"=w320) -> ()  [unwired: 1 in, 1 out]
    n170 = xnode "2"("Duty Cycle"=w319) -> ()  [unwired: 1 in, 1 out]
    n171 = Divide(x=0.32, y=200) -> (x/y=w347:dbl)
    n172 = Divide(x=0.32, y=200) -> (x/y=w352:dbl)
    n173 = Multiply(x=w311, y=w347) -> (x*y=w346:dbl)
    n174 = Multiply(x=w314, y=w352) -> (x*y=w351:dbl)
    n175 = Add(x=w346, y=0.6) -> (x+y=→"thruster 2":dbl)
    n176 = Add(x=w351, y=0.6) -> (x+y=→"thruster 1":dbl)
    n177 = local write "yav"(w356) -> ()
    n178 = local write "surd"(w358) -> ()
    n179 = local write "yad"(w359) -> ()
    n180 = local write "surv"(w357) -> ()
    n181 = xnode "LED"("LED2"=TRUE) -> ()  [unwired: 1 in, 1 out]
  }
  n182 = UDP Close(connection ID=w2, 8:w1) -> ()  [unwired: 2 out]
  n183 = UDP Close(connection ID=w7, 8:w6) -> ()  [unwired: 2 out]
  n184 = UDP Close(connection ID=w11, 8:w12) -> ()  [unwired: 2 out]
